vi "Show name.vi"(8 "error in (no error)":errorcluster, 11 "Mag Lab Measure Base in":refnum<class "Mag Lab Measure Base.lvclass">) -> (0 "error out":errorcluster, 3 "Mag Lab Measure Base out":refnum<class "Mag Lab Measure Base.lvclass">)   [LabVIEW 2015, in "Mag Lab Measure Base.lvclass"]
uses:
  Mag Lab Measure Base.lvclass
  Mag Lab Root/Mag Lab Root.lvclass/Mag Lab Root.ctl
  Mag Lab Measure Base.lvclass/Mag Lab Measure Base.ctl
  Mag Lab Root/Mag Lab Root.lvclass
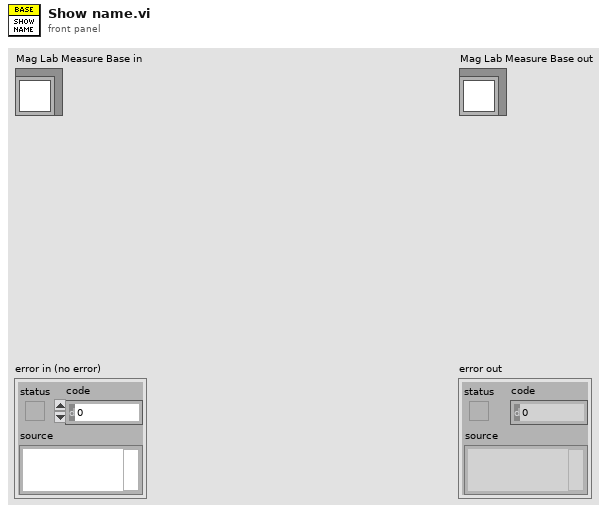
[diagram p1: front panel]
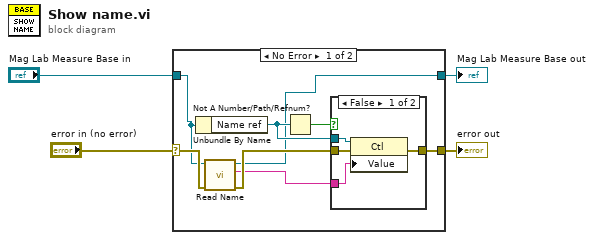
[diagram p0: block diagram]
diagram:
  n1 = case shown="No Error" "error in (no error)" {
    selector: "error in (no error)" -> [w9 w19]
    tunnel: [w10 w19] -> w3
    tunnel: [w6 w18] -> w1
    tunnel: "Mag Lab Measure Base in" -> [w7 w18]
    frame No Error {
      n2 = Unbundle By Name(w7) -> ("Name ref"=w11:refnum<vi>)
      n3 = call "Read Name.vi"("error in (no error)"=w9, "Mag Lab Root in"=w7) -> ("error out"=w8:errorcluster, "Name"=w5:string, "Mag Lab Root out"=w6:refnum<class "Mag Lab Measure Base.lvclass">)  [unwired: 7 in]
      n4 = Not A Number/Path/Refnum?(number/path/refnum=w11) -> (NaN/Path/Refnum?=w12:bool)
      n5 = case shown="False" w12 {
        tunnel: w11 -> [w16 _]
        tunnel: w5 -> [w15 _]
        tunnel: w8 -> [w14 w17]
        tunnel: [w13 w17] -> w10
        frame False {
          n6 = property class="Ctl"(reference=w16, error in=w14, "Value"=w15) -> (error out=w13:errorcluster)  [unwired: 1 out]
        }
        frame True {
        }
      }
    }
    frame Error {
    }
  }
  "error out" <- w3
  "Mag Lab Measure Base out" <- w1
